vi "FullAlign.vi"(0 "Joystick 0":dbl, 1 "Joystick 1":dbl, 4 "Distance":dbl=21.792199999999994, 5 "Angle":dbl=-43.59074216711602, 8 "Button":bool=TRUE) -> (20 "Right Motor":dbl, 21 "Left Motor":dbl=-0.0, 25 "Not In Sight?":bool=TRUE, 27 "In Range?":bool=TRUE)   [LabVIEW 2016]
uses:
  Systems/Global 1.vi
panel:
  in  "Forward Speed":dbl format="%#_13g"
  in  "Max Error":dbl=100.0 format="%#_13g"
  in  "Turn_Gain":dbl=0.25 format="%#_13g"
  in  "Align Effort Addition":dbl=0.175 min=0.0 max=1.0 step=0.05 format="%#_13g"
  in  "Align Target":dbl format="%#_13g"
  in  "MinDistance":dbl=24.0 format="%#_13g"
  out "Sees Target?":bool=TRUE
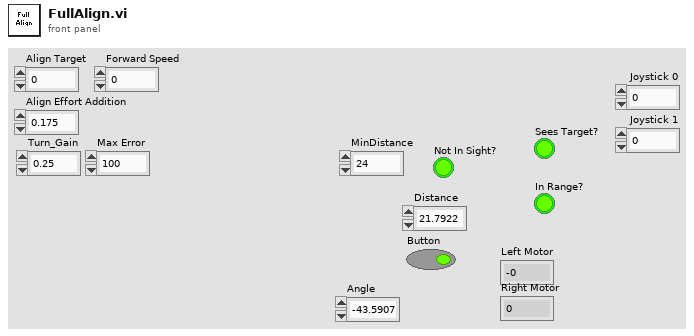
[diagram p1: front panel]
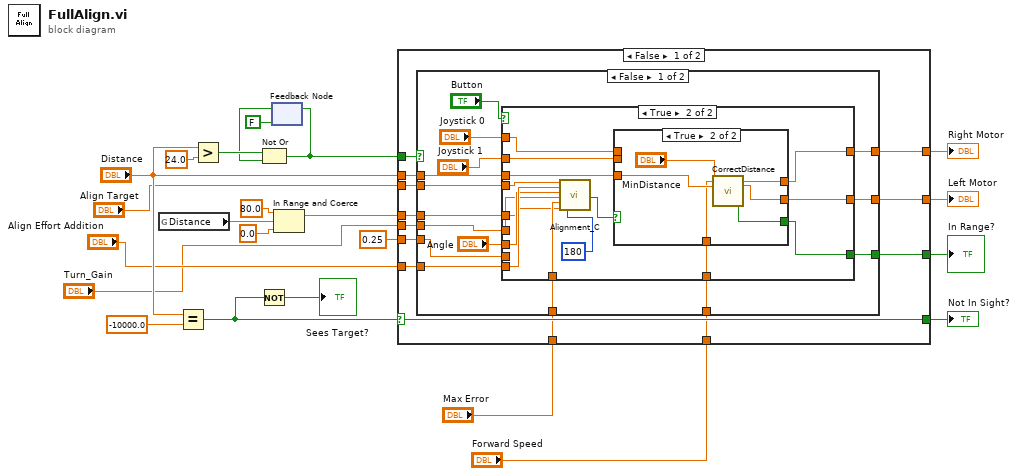
[diagram p0: block diagram]
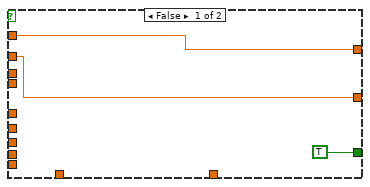
[diagram p2: hidden frame]
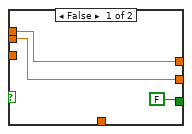
[diagram p3: hidden frame]
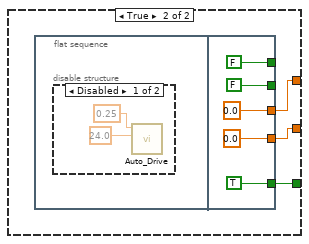
[diagram p4: hidden frame]
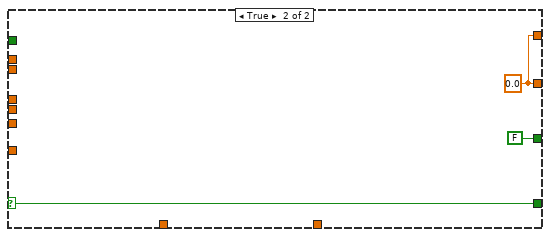
[diagram p6: hidden frame]
diagram:
  n1 = global read "Global 1.vi" "Distance"() -> (w10:dbl)
  n2 = Equal?(x="Distance", y=-10000.0) -> (x = y?=w11:bool)
  n3 = Greater?(x="Distance", y=24.0) -> (0:w16:bool)
  n4 = Not(x=w11) -> (.not. x?=→"Sees Target?":bool)
  n5 = feedback #1(FALSE) -> (w15:bool)
  n6 = Not Or(1:w15, 2:w16) -> (0:w17:bool)
  n7 = feedback-in #1(w17) -> ()
  n8 = In Range and Coerce(upper limit=80.0, x=w10, lower limit=0.0) -> (coerced(x)=w7:dbl)  [unwired: 1 out]
  n9 = case shown="False" w11 {
    selector: w11 -> [w29 w89]
    tunnel: w17 -> [w36 _]
    tunnel: [w35 w90] -> w22
    tunnel: [w34 w90] -> w12
    tunnel: [w33 FALSE] -> w18
    tunnel: "Distance" -> [w32 _]
    tunnel: 0.25 -> [w31 _]
    tunnel: w7 -> [w30 _]
    tunnel: [w29 w89] -> w6
    tunnel: "Align Target" -> [w28 _]
    tunnel: "Align Effort Addition" -> [w27 _]
    tunnel: "Turn_Gain" -> [w26 _]
    tunnel: "Max Error" -> [w25 _]
    tunnel: "Forward Speed" -> [w24 _]
    frame False {
      n10 = case shown="False" w36 {
        tunnel: w32 -> [w47 _]
        tunnel: [w46 w80] -> w35
        tunnel: [w45 w79] -> w34
        tunnel: [w44 w81] -> w33
        tunnel: w31 -> [w43 _]
        tunnel: w30 -> [w42 _]
        tunnel: w28 -> [w41 _]
        tunnel: w27 -> [w40 _]
        tunnel: w26 -> [w39 _]
        tunnel: w25 -> [w38 _]
        tunnel: w24 -> [w37 _]
        frame False {
          n11 = case shown="True" "Button" {
            tunnel: "Joystick 1" -> [w53 w57]
            tunnel: "Joystick 0" -> [w54 w56]
            tunnel: [w53 w69] -> w45
            tunnel: [w54 w68] -> w46
            tunnel: "Angle" -> [_ w63]
            tunnel: [TRUE w67] -> w44
            tunnel: w47 -> [_ w66]
            tunnel: w43 -> [_ _]
            tunnel: w42 -> [_ w59]
            tunnel: w41 -> [_ w65]
            tunnel: w40 -> [_ w64]
            tunnel: w39 -> [_ w62]
            tunnel: w38 -> [_ w61]
            tunnel: w37 -> [_ w55]
            frame False {
            }
            frame True {
              n12 = call "Alignment_C.vi"("Target"=w65, "Effort Addition"=w64, "Camera Feedback"=w63, "Turn_Gain"=w62, "Max Error"=w61, "Range"=w59, "POV"=180) -> ("LeftAndRight?"=w58:bool)  [unwired: 12 in]
              n13 = case shown="True" w58 {
                tunnel: [w71 w77] -> w69
                tunnel: [w70 w76] -> w68
                tunnel: [FALSE w74] -> w67
                tunnel: w66 -> [_ w75]
                tunnel: w57 -> [w71 _]
                tunnel: w56 -> [w70 _]
                tunnel: w55 -> [_ w73]
                frame False {
                }
                frame True {
                  n14 = call "CorrectDistance.vi"("Speed"=w73, "CenterPoint"="MinDistance", "Distance"=w75) -> ("In Range?"=w74:bool, "Right Motor"=w76:dbl, "Left Motor"=w77:dbl)  [unwired: 22 in]
                }
              }
            }
          }
        }
        frame True {
          n15 = flat-sequence {
            tunnel: [FALSE] -> _
            tunnel: [FALSE] -> _
            tunnel: [TRUE] -> w81
            tunnel: [0.0] -> w80
            tunnel: [0.0] -> w79
            frame #0 {
              n16 = disable-structure shown="Disabled" {
                frame Disabled {
                  n17 = call "Auto_Drive.vi"("distance"=24.0, "Drive Effort"=0.25) -> ()  [unwired: 10 in]
                }
                frame Enabled {
                }
              }
            }
            frame #1 {
            }
          }
        }
      }
    }
    frame True {
      w90 = 0.0
    }
  }
  "Right Motor" <- w22
  "Left Motor" <- w12
  "In Range?" <- w18
  "Not In Sight?" <- w6
